vi "Modbus_Master.vi"() -> ()   [LabVIEW 2020]
uses:
  <vilib>/NI/Modbus Library/API/Wrapper/Create TCP Master.vi
  <vilib>/NI/Modbus Library/API/Master/Modbus Master.lvclass
  <vilib>/NI/Modbus Library/API/Wrapper/API Main.lvlib
panel:
  in  "Array":u16[](array[slide]) scale=0.0..100.0
  in  "address 2":u16
  in  "Thermometer":u16(slide) scale=0.0..100.0
  in  "address":u16
  in  "stop":bool
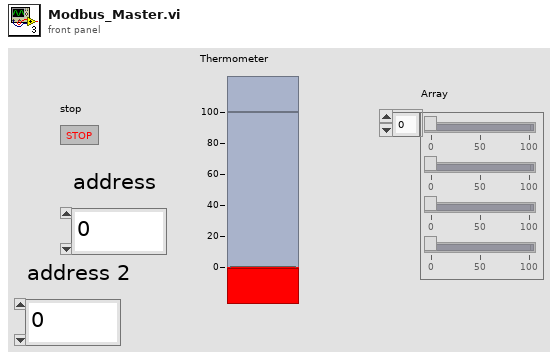
[diagram p1: front panel]
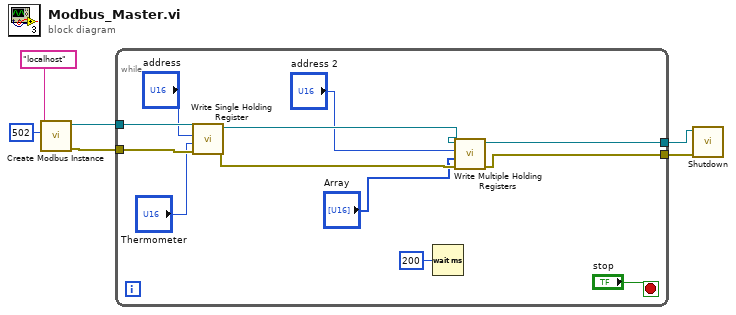
[diagram p0: block diagram]
diagram:
  n1 = call-poly <vilib>:"Create Modbus Instance.vi"("port (502)"=u16 502, "address"="localhost") -> ("error out"=w3:errorcluster, "TCP master instance"=w4:refnum<class "Modbus Master.lvclass">)  [unwired: 8 in]
  n2 = while {
    tunnel: w4 -> [w17]
    tunnel: w3 -> [w16]
    tunnel: [w11] -> w2
    tunnel: [w10] -> w1
    stop <- "stop" stop-if-true
    n3 = call-dynamic "Write Single Holding Register.vi"("error in"=w16, "register to write"="Thermometer", "address"="address", "Modbus master in"=w17) -> ("error out"=w9:errorcluster, "Modbus master out"=w12:refnum<class "Modbus Master.lvclass">)  [unwired: 6 in]
    n4 = Wait (ms)(milliseconds to wait=u32 200) -> ()  [unwired: 1 out]
    n5 = call-dynamic "Write Multiple Holding Registers.vi"("error in"=w9, "registers to write"="Array", "starting address"="address 2", "Modbus master in"=w12) -> ("error out"=w10:errorcluster, "Modbus master out"=w11:refnum<class "Modbus Master.lvclass">)  [unwired: 6 in]
  }
  n6 = call-dynamic "Shutdown.vi"("error in"=w1, "Modbus master in"=w2) -> ()  [unwired: 9 in, 1 out]
